vi "EXPERIMENTAL_RECONFIGURE_OSCOPE_CARD_JSON.vi"() -> ()   [LabVIEW 2019]
uses:
  <instrlib>/niScope/Controls/niScope vertical coupling.ctl
  Controls/OscilloscopeBlockControl2.ctl
  <instrlib>/niScope/Configure/Trigger/niScope Configure Trigger Software.vi
  Controls/OscilloscopeBlockControl.ctl
panel:
  in  "Oscilloscope Block Parameters":T1={"Oscilloscope"="", "channel names list"="", "vertical range"=10.0, "vertical coupling"=1, "Channel 0 50 ohms?"=FALSE, "50 ohm vertical range (V)"=10.0, "min record length"=1000, "min sample rate"=20000000.0} {"min sample rate" format="%^.2e"; "vertical coupling" items=["AC", "DC", "Ground"]}
  out "Array":T3(array[cluster]) {"vertical coupling" items=["AC", "DC", "Ground"]}
  in  "Exit to Collection":bool
  in  "Oscilloscope Block":T1={"Oscilloscope"="", "channel names list"="", "vertical range"=10.0, "vertical coupling"=1, "Channel 0 50 ohms?"=FALSE, "50 ohm vertical range (V)"=10.0, "min record length"=1000, "min sample rate"=20000000.0} {"min sample rate" format="%^.2e"; "vertical coupling" items=["AC", "DC", "Ground"]}
  in  "apply changes":bool
  out "output cluster":T4 {"vertical coupling" items=["AC", "DC", "Ground"]}
  out "Oscilloscope Configuration Input Array":T4[](array[typedef]) {"vertical coupling" items=["AC", "DC", "Ground"]}
  in  "JSON String":string
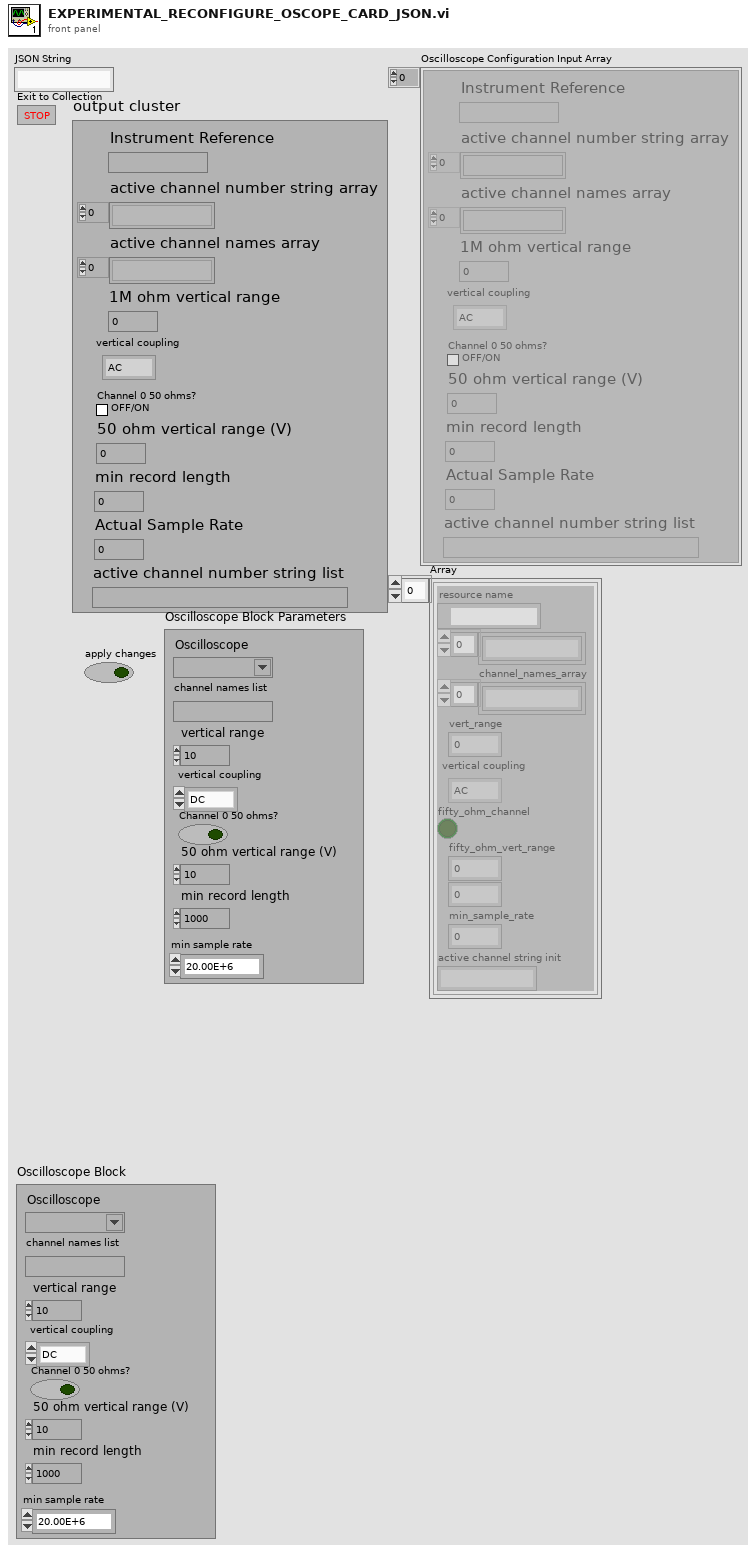
[diagram p1: front panel]
types:
  T1 = typedef "OscilloscopeBlockControl.ctl" = cluster{"Oscilloscope":refnum<k15>, "channel names list":string, "vertical range":dbl, "vertical coupling":T2, "Channel 0 50 ohms?":bool, "50 ohm vertical range (V)":dbl, "min record length":i32, "min sample rate":dbl}
  T2 = typedef "niScope vertical coupling.ctl" = i32
  T3 = cluster{"resource name":refnum<k15>, string[], "channel_names_array":string[], "vert_range":dbl, "vertical coupling":T2, "fifty_ohm_channel":bool, "fifty_ohm_vert_range":dbl, i32, "min_sample_rate":dbl, "active channel string init":string}[]
  T4 = typedef "OscilloscopeBlockControl2.ctl" = cluster{"Instrument Reference":refnum<k15>, "active channel number string array":string[], "active channel names array":string[], "1M ohm vertical range":dbl, "vertical coupling":T2, "Channel 0 50 ohms?":bool, "50 ohm vertical range (V)":dbl, "min record length":i32, "Actual Sample Rate":dbl, "active channel number string list":string}
  T5 = cluster{"Oscilloscope_Number":dbl, "Oscilloscope_Array":cluster{"oscope_instr_name":string, "channel_names_array":string[], "vert_range":dbl, "coupling":string, "fifty_ohm_channel":bool, "fifty_ohm_vert_range":dbl, "min_record_length":dbl, "min_sample_rate":dbl}[]}
  T6 = cluster{"oscope_instr_name":string, "channel_names_array":string[], "vert_range":dbl, "coupling":string, "fifty_ohm_channel":bool, "fifty_ohm_vert_range":dbl, "min_record_length":dbl, "min_sample_rate":dbl}[]
  T7 = cluster{"resource name":refnum<k15>, string[], "channel_names_array":string[], "vert_range":dbl, "vertical coupling":T2, "fifty_ohm_channel":bool, "fifty_ohm_vert_range":dbl, i32, "min_sample_rate":dbl, "active channel string init":string}
  T8 = cluster{"resource name":refnum<k15>, "active channel string init":string, "vert_range":dbl, "vertical coupling":T2, "fifty_ohm_channel":bool, "fifty_ohm_vert_range":dbl, i32, "min_sample_rate":dbl}
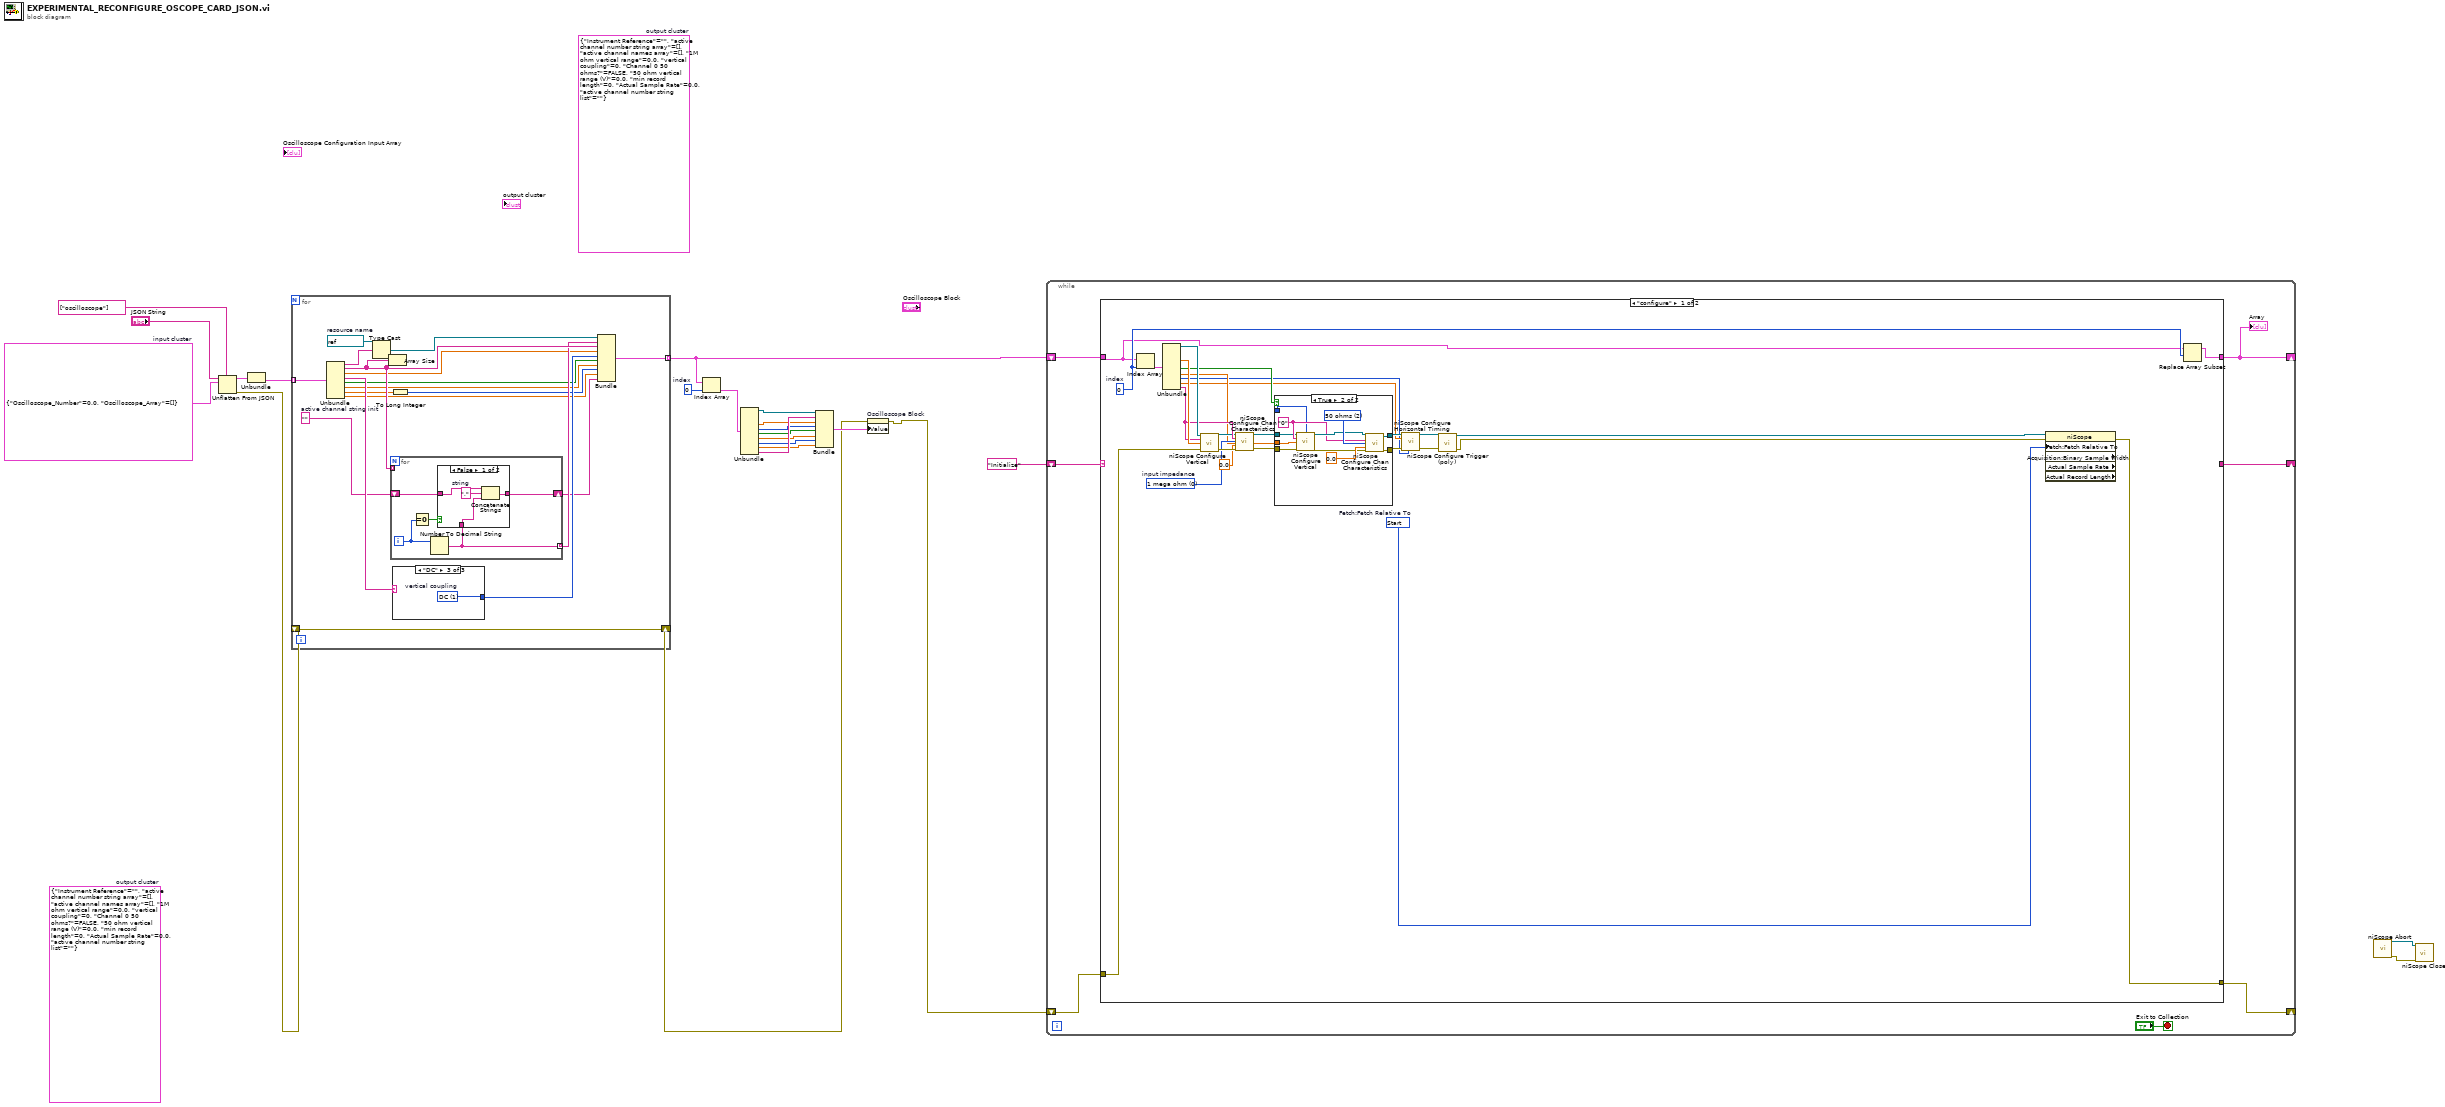
[diagram p0: block diagram]
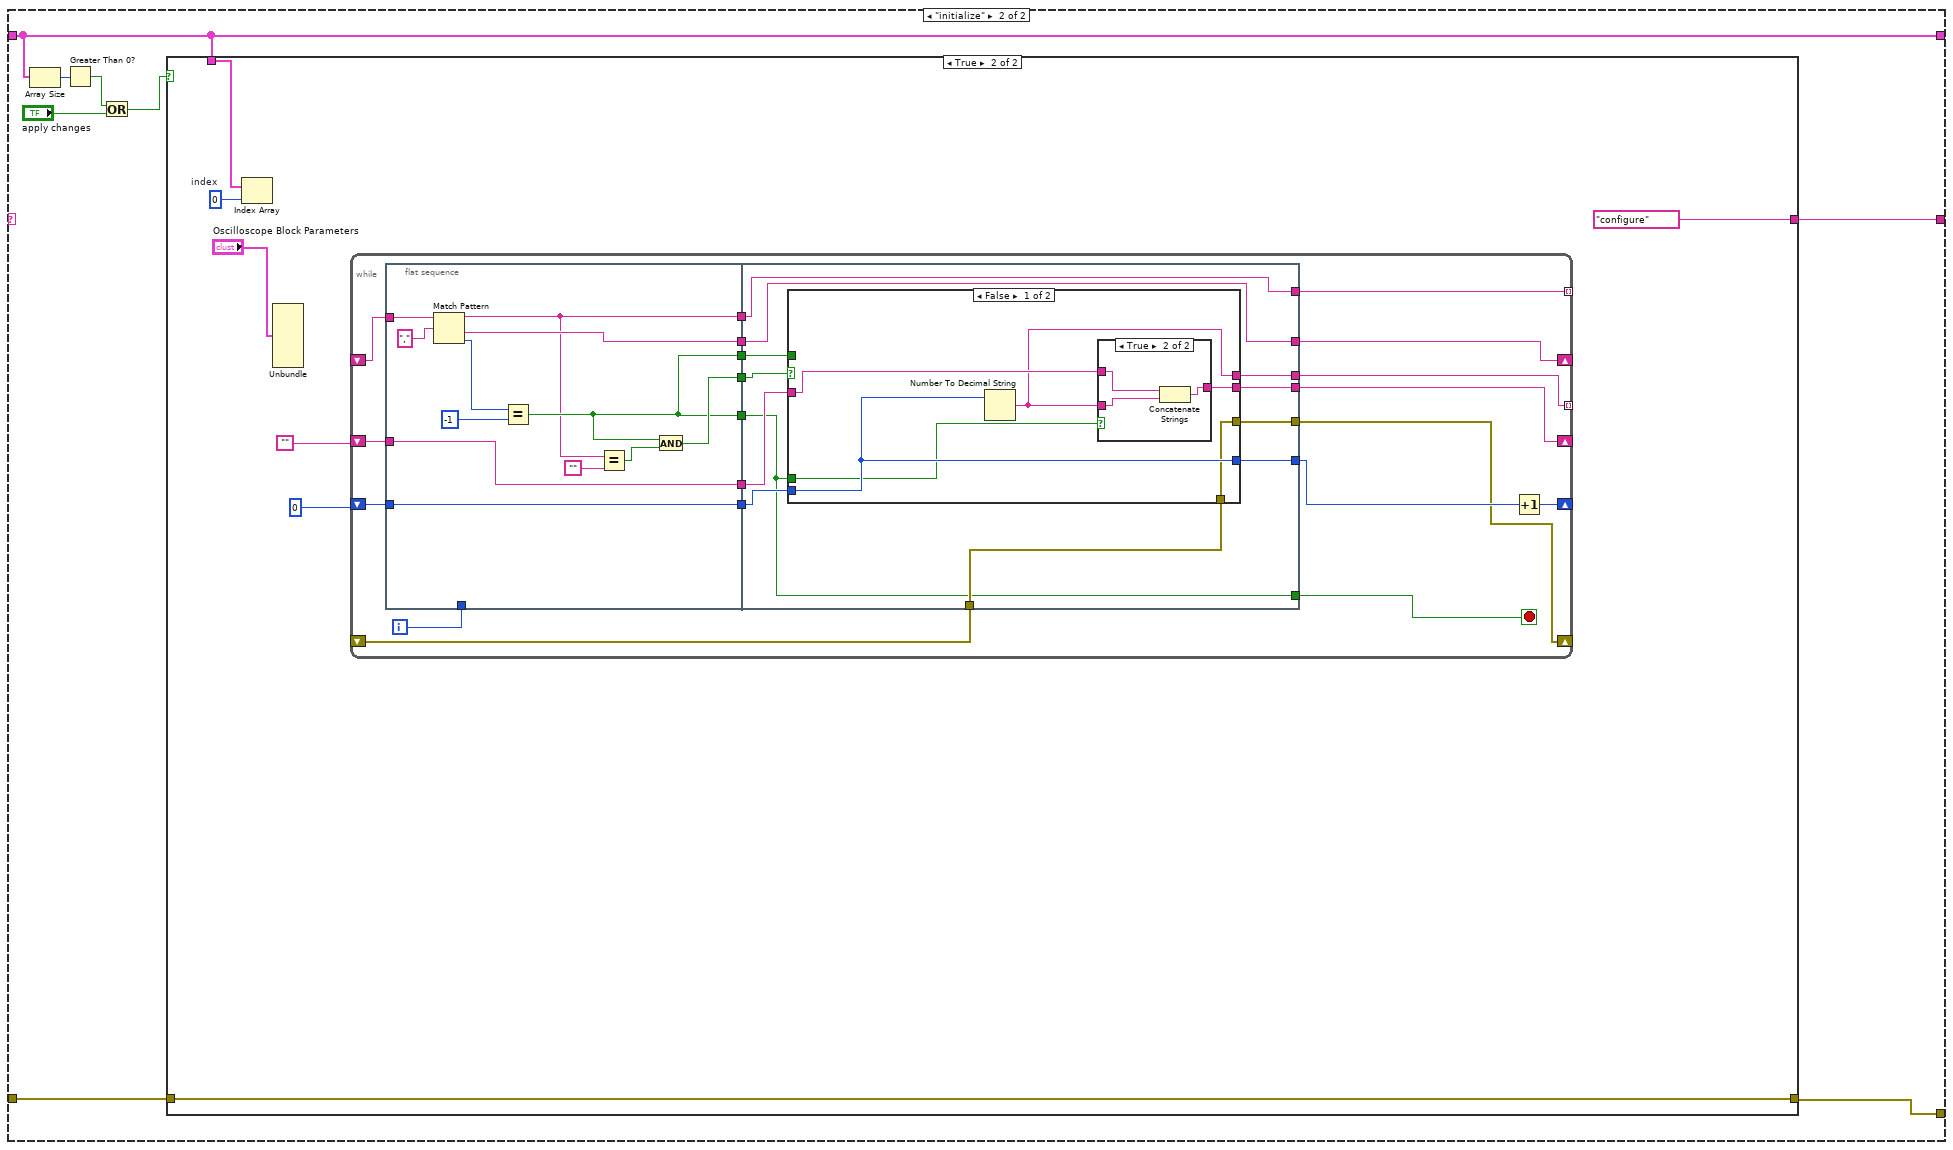
[diagram p3: hidden frame]
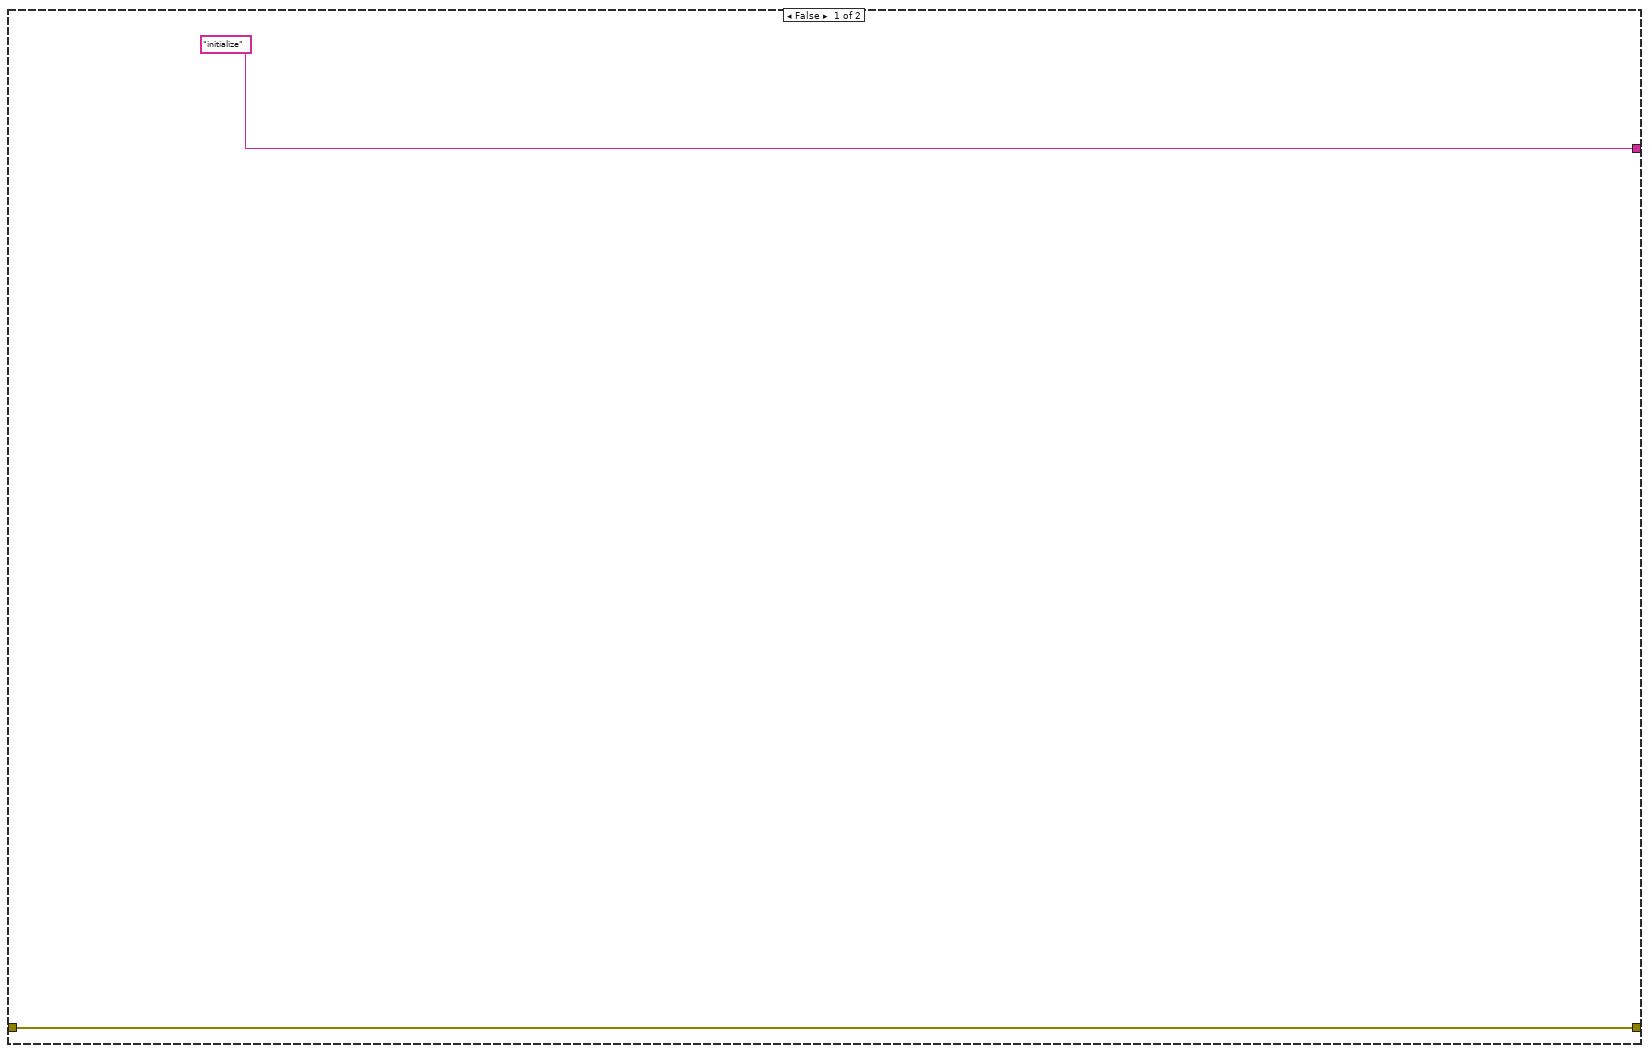
[diagram p4: hidden frame]
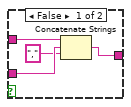
[diagram p5: hidden frame]
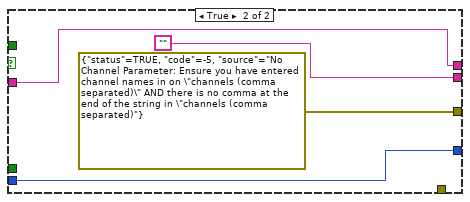
[diagram p6: hidden frame]
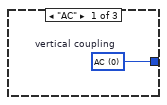
[diagram p8: hidden frame]
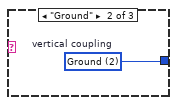
[diagram p9: hidden frame]
diagram:
  w15 = 0  # index
  (unwired) T4 {"Instrument Reference"="", "active channel number string array"=[], "active channel names array"=[], "1M ohm vertical range"=0.0, "vertical coupling"=0, "Channel 0 50 ohms?"=FALSE, "50 ohm vertical range (V)"=0.0, "min record length"=0, "Actual Sample Rate"=0.0, "active channel number string list"=""}  # output cluster
  (unwired) T4 {"Instrument Reference"="", "active channel number string array"=[], "active channel names array"=[], "1M ohm vertical range"=0.0, "vertical coupling"=0, "Channel 0 50 ohms?"=FALSE, "50 ohm vertical range (V)"=0.0, "min record length"=0, "Actual Sample Rate"=0.0, "active channel number string list"=""}  # output cluster
  w21 = T5 {"Oscilloscope_Number"=0.0, "Oscilloscope_Array"=[]}  # input cluster
  n1 = Unflatten From JSON(path=string[] ["oscilloscope"], JSON string="JSON String", type and defaults=w21) -> (value=w20:T5, error out=w5:errorcluster)  [unwired: 4 in]
  n2 = Unbundle(w20) -> ("Oscilloscope_Array"=w19:T6)  [unwired: 1 out]
  n3 = for {
    tunnel: w19 -> [w41] mode=indexing
    tunnel: [w25] -> w17 mode=indexing
    shift-right: [w24] -> w4
    shift-left: w5 -> [w24]
    w37 = ""  # active channel string init
    w40 = refnum<k15> refnum  # resource name
    n4 = Unbundle(w41) -> ("oscope_instr_name"=w39:string, "channel_names_array"=w35:string[], "vert_range"=w33:dbl, "coupling"=w38:string, "fifty_ohm_channel"=w31:bool, "fifty_ohm_vert_range"=w30:dbl, "min_record_length"=w29:dbl, "min_sample_rate"=w27:dbl)
    n5 = Type Cast(type=w40, x=w39) -> (*(type *) &x=w36:refnum<k15>)
    n6 = Array Size(array=w35) -> ()  [unwired: 1 out]
    n7 = for {
      tunnel: w35 -> [_] mode=indexing
      tunnel: [w44] -> w34 mode=indexing
      shift-right: [w43] -> w26
      shift-left: w37 -> [w42]
      i -> [w46]
      n8 = Equal To 0?(x=w46) -> (x = 0?=w45:bool)
      n9 = Number To Decimal String(number=w46) -> (decimal integer string=w44:string)  [unwired: 1 in]
      n10 = case shown="False" w45 {
        tunnel: w44 -> [w47 w51]
        tunnel: w42 -> [w49 _]
        tunnel: [w50 w51] -> w43
        frame False {
          w48 = ","  # string
          n11 = Concatenate Strings(w49, w48, w47) -> (w50:string)
        }
        frame True {
        }
      }
    }
    n12 = To Long Integer(number=w29) -> (32bit integer=w28:i32)
    n13 = case shown="\"DC\"" w38 {
      tunnel: [w52 w53 w54] -> w32
      frame "AC" {
        w52 = T2 0 items=["AC", "DC", "Ground"]  # vertical coupling
      }
      frame "Ground" {
        w53 = T2 2 items=["AC", "DC", "Ground"]  # vertical coupling
      }
      frame "DC" {
        w54 = T2 1 items=["AC", "DC", "Ground"]  # vertical coupling
      }
    }
    n14 = Bundle("resource name"=w36, w34, "channel_names_array"=w35, "vert_range"=w33, "vertical coupling"=w32, "fifty_ohm_channel"=w31, "fifty_ohm_vert_range"=w30, w28, "min_sample_rate"=w27, "active channel string init"=w26) -> (w25:T7)  [unwired: 1 in]
  }
  n15 = Index Array(array=w17, index=w15) -> (element=w14:T7)
  n16 = Unbundle(w14) -> ("resource name"=w13:refnum<k15>, "vert_range"=w11:dbl, "vertical coupling"=w10:T2, "fifty_ohm_channel"=w9:bool, "fifty_ohm_vert_range"=w8:dbl, w7:i32, "min_sample_rate"=w6:dbl, "active channel string init"=w12:string)  [unwired: 2 out]
  n17 = Bundle("resource name"=w13, "active channel string init"=w12, "vert_range"=w11, "vertical coupling"=w10, "fifty_ohm_channel"=w9, "fifty_ohm_vert_range"=w8, w7, "min_sample_rate"=w6) -> (w16:T8)  [unwired: 1 in]
  n18 = property on="Oscilloscope Block" class="Clust (strict)"(error in=w4, "Value"=w16) -> (error out=w3:errorcluster)  [unwired: 1 in, 1 out]
  n19 = while {
    shift-right: [w58] -> _
    shift-left: w17 -> [w60]
    shift-right: [w59] -> _
    shift-left: "Initialize" -> [w61]
    shift-right: [w55] -> _
    shift-left: w3 -> [w56]
    stop <- "Exit to Collection" stop-if-true
    n20 = case shown="\"configure\"" w61 {
      tunnel: w60 -> [w62 w102]
      tunnel: [_ w108] -> w59
      tunnel: [w63 w102] -> w58
      tunnel: w56 -> [w86 w104]
      tunnel: [w66 w103] -> w55
      frame "configure" {
        w64 = 482 items=["Start"=482, "Trigger"=483, "Pretrigger"=477, "Now"=481, "Read Pointer"=388]  # Fetch:Fetch Relative To
        w82 = u32 0 items=["1 mega ohm"=0, "50 ohms"=2]  # input impedance
        w65 = 0  # index
        n21 = Index Array(array=w62, index=w65) -> (element=w85:T7)
        n22 = Unbundle(w85) -> ("resource name"=w84:refnum<k15>, "vert_range"=w83:dbl, "fifty_ohm_channel"=w79:bool, "fifty_ohm_vert_range"=w76:dbl, w70:i32, "min_sample_rate"=w71:dbl, "active channel string init"=w81:string)  [unwired: 3 out]
        n23 = call <instrlib>:"niScope Configure Vertical.vi"("instrument handle"=w84, "channels"=w81, "vertical range"=w83, "error in"=w86) -> ("instrument handle out"=w80:refnum<k15>, "error out"=w88:errorcluster)  [unwired: 10 in]
        n24 = call <instrlib>:"niScope Configure Chan Characteristics.vi"("instrument handle"=w80, "channels"=w81, "input impedance"=w82, "maximum input frequency"=0.0, "error in"=w88) -> ("instrument handle out"=w78:refnum<k15>, "error out"=w77:errorcluster)  [unwired: 9 in]
        n25 = case shown="True" w79 {
          tunnel: [w90 w101] -> w72
          tunnel: [w89 w100] -> w74
          tunnel: w78 -> [w90 w94]
          tunnel: w77 -> [w89 w93]
          tunnel: _ -> [_ w92]
          tunnel: w76 -> [_ w91]
          frame False {
          }
          frame True {
            w98 = u32 2 items=["1 mega ohm"=0, "50 ohms"=2] ("input impedance")
            w95 = "0" ("channels")
            n26 = call <instrlib>:"niScope Configure Vertical.vi"("instrument handle"=w94, "vertical coupling"=w92, "channels"=w95, "vertical range"=w91, "error in"=w93) -> ("instrument handle out"=w97:refnum<k15>, "error out"=w96:errorcluster)  [unwired: 9 in]
            n27 = call <instrlib>:"niScope Configure Chan Characteristics.vi"("instrument handle"=w97, "channels"=w95, "input impedance"=w98, "maximum input frequency"=0.0, "error in"=w96) -> ("instrument handle out"=w101:refnum<k15>, "error out"=w100:errorcluster)  [unwired: 9 in]
          }
        }
        n28 = call <instrlib>:"niScope Configure Horizontal Timing.vi"("instrument handle"=w72, "min sample rate"=w71, "error in"=w74, "min record length"=w70) -> ("instrument handle out"=w75:refnum<k15>, "error out"=w73:errorcluster)  [unwired: 10 in]
        n29 = call-poly <instrlib>:"niScope Configure Trigger (poly).vi"("instrument handle"=w75, "error in"=w73) -> ("instrument handle out"=w68:refnum<k15>, "error out"=w67:errorcluster)  [unwired: 12 in]
        n30 = property class="niScope" props=["Fetch:Fetch Relative To", "Acquisition:Binary Sample Width", "Actual Sample Rate", "Actual Record Length"](reference=w68, error in=w67, "Fetch:Fetch Relative To"=w64) -> (error out=w66:errorcluster, "Actual Record Length"=w69:i32)  [unwired: 3 out]
        n31 = Replace Array Subset(array=w62, index=w65) -> (w63:T3)  [unwired: 1 in]
      }
      frame "initialize" {
        n32 = Array Size(array=w102) -> (size(s)=w109:i32)
        n33 = Greater Than 0?(x=w109) -> (x > 0?=w107:bool)
        n34 = Or(x=w107, y="apply changes") -> (x .or. y?=w105:bool)
        n35 = case shown="True" w105 {
          tunnel: ["initialize" "configure"] -> w108
          tunnel: w104 -> [w110 w117]
          tunnel: [w110 w117] -> w103
          tunnel: w102 -> [_ w114]
          frame False {
          }
          frame True {
            w113 = 0  # index
            n36 = Index Array(array=w114, index=w113) -> ()  [unwired: 1 out]
            n37 = Unbundle("Oscilloscope Block Parameters") -> ()  [unwired: 8 out]
            n38 = while {
              shift-right: [w137] -> _
              shift-left: _ -> [w138]
              shift-right: [w125] -> _
              shift-left: 0 -> [w130]
              shift-right: [w122] -> _
              shift-left: "" -> [w128]
              tunnel: [w121] -> _ mode=indexing
              shift-right: [w123] -> _
              shift-left: _ -> [w127]
              tunnel: [w119] -> _ mode=indexing
              i -> [w136]
              stop <- w135 stop-if-true
              n39 = flat-sequence {
                tunnel: w138 -> [w148]
                tunnel: w136 -> [_]
                tunnel: [w146] -> w134
                tunnel: [w140] -> w133
                tunnel: [w141] -> w132
                tunnel: [w145] -> w131
                tunnel: w130 -> [w145]
                tunnel: [w144] -> w129
                tunnel: w128 -> [w144]
                tunnel: [w140] -> w124
                tunnel: [w139] -> w120
                tunnel: w134 -> [w162]
                tunnel: w133 -> [w153]
                tunnel: w132 -> [w161]
                tunnel: w131 -> [w159]
                tunnel: w129 -> [w158]
                tunnel: w127 -> [w157]
                tunnel: [w162] -> w137
                tunnel: [w153] -> w135
                tunnel: [w160] -> w122
                tunnel: [w156] -> w123
                tunnel: [w155] -> w126
                tunnel: w124 -> [w154]
                tunnel: [w152] -> w121
                tunnel: w120 -> [w152]
                tunnel: [w151] -> w119
                frame #0 {
                  n40 = Match Pattern(string=w148, regular expression=",") -> (before substring=w139:string, after substring=w146:string, offset past match=w150:i32)  [unwired: 1 in, 1 out]
                  n41 = Equal?(x=w150, y=-1) -> (x = y?=w140:bool)
                  n42 = Equal?(x=w139, y="") -> (x = y?=w142:bool)
                  n43 = And(x=w140, y=w142) -> (x .and. y?=w141:bool)
                }
                frame #1 {
                  n44 = case shown="False" w161 {
                    tunnel: [w164 ""] -> w160
                    tunnel: w159 -> [w168 w178]
                    tunnel: w158 -> [w166 w176]
                    tunnel: [w168 w178] -> w155
                    tunnel: w157 -> [w167 _]
                    tunnel: [w167 errorcluster {"status"=TRUE, "code"=-5, "source"="No Channel Parameter: Ensure you have entered channel names in on \"channels (comma separated)\" AND there is no comma at the end of the string in \"channels (comma separated)"} ("error out")] -> w156
                    tunnel: w154 -> [_ _]
                    tunnel: w153 -> [w165 _]
                    tunnel: [w163 w176] -> w151
                    frame False {
                      n45 = Number To Decimal String(number=w168) -> (decimal integer string=w163:string)  [unwired: 1 in]
                      n46 = case shown="True" w165 {
                        tunnel: w166 -> [w172 w175]
                        tunnel: w163 -> [w171 w174]
                        tunnel: [w169 w173] -> w164
                        frame False {
                          n47 = Concatenate Strings(w172, w171, "," ("string")) -> (w169:string)
                        }
                        frame True {
                          n48 = Concatenate Strings(w175, w174) -> (w173:string)
                        }
                      }
                    }
                    frame True {
                    }
                  }
                }
              }
              n49 = Increment(x=w126) -> (x+1=w125:i32)
            }
          }
        }
      }
    }
    "Array" <- w58
  }
  n50 = call <instrlib>:"niScope Abort.vi"() -> ("instrument handle out"=w1:refnum<k15>, "error out"=w2:errorcluster)  [unwired: 14 in]
  n51 = call <instrlib>:"niScope Close.vi"("instrument handle"=w1, "error in"=w2) -> ()  [unwired: 13 in, 1 out]
